vi "RecibirParametros.vi"(8 "error in (no error)":errorcluster, 10 "Parametros":T1, 11 "Measurement Señal Actualizable in":refnum<class "Measurement Señal Actualizable.lvclass">) -> (0 "error out":errorcluster, 3 "Measurement Señal Actualizable out":refnum<class "Measurement Señal Actualizable.lvclass">)   [LabVIEW 2020, in "Measurement Señal Actualizable.lvlib" / "Measurement Señal Actualizable.lvclass"]
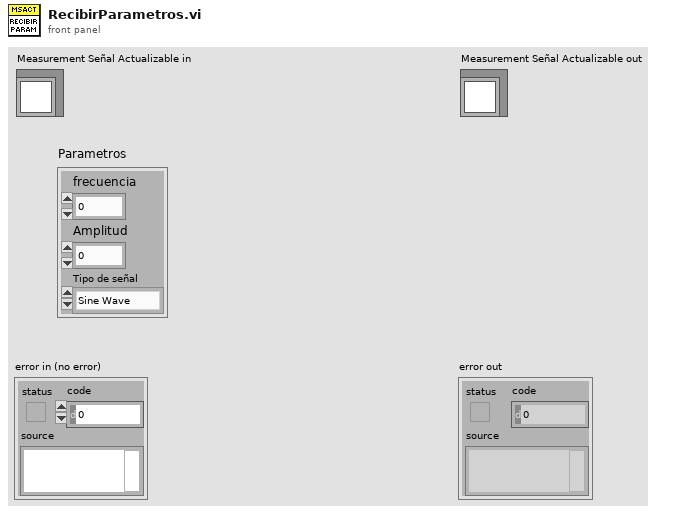
[diagram p1: front panel]
types:
  T1 = cluster{"frecuencia":dbl, "Amplitud":dbl, "Tipo de señal":enum16{"Sine Wave", "Triangle Wave", "Square Wave", "Sawtooth Wave"}}
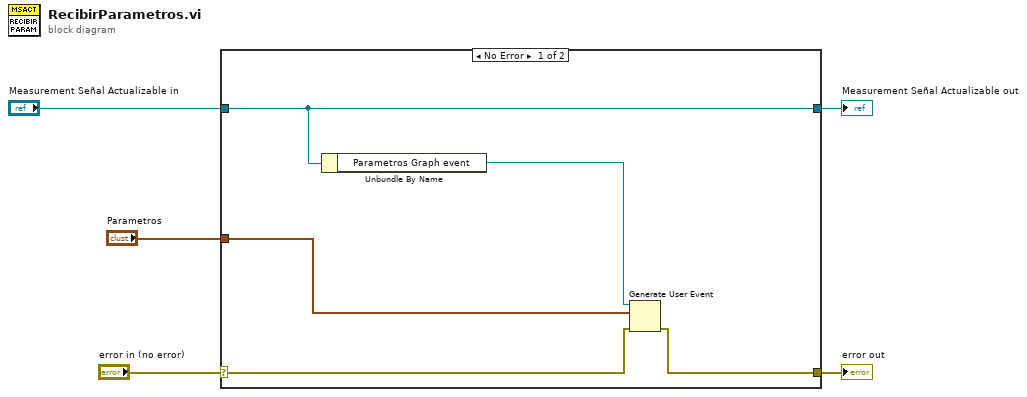
[diagram p0: block diagram]
diagram:
  n1 = case shown="No Error" "error in (no error)" {
    selector: "error in (no error)" -> [w8 w12]
    tunnel: [w9 w12] -> w4
    tunnel: [w10 w11] -> w2
    tunnel: "Measurement Señal Actualizable in" -> [w10 w11]
    tunnel: "Parametros" -> [w6 _]
    frame No Error {
      n2 = Unbundle By Name(w10) -> ("Parametros Graph event"=w7:refnum<user-event>)
      n3 = Generate User Event(user event=w7, event data cluster=w6, error in=w8) -> (error out=w9:errorcluster)  [unwired: 1 in, 1 out]
    }
    frame Error {
    }
  }
  "error out" <- w4
  "Measurement Señal Actualizable out" <- w2
